vi "Access File Compress Database.vi"(8 "error in":errorcluster caption="error in (no error)", 11 "Access File Path":path caption="Access File Path (*.mdb)") -> (0 "error out":errorcluster)   [LabVIEW 2014]
panel:
  # "Input"
  # "Local"
  # "Output"
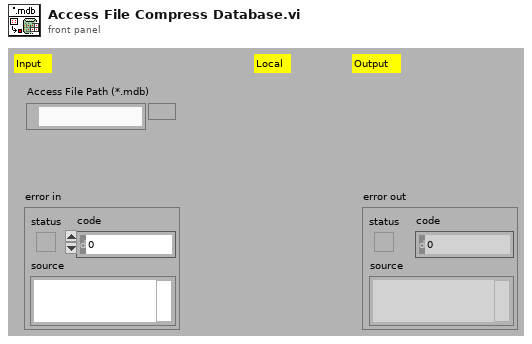
[diagram p1: front panel]
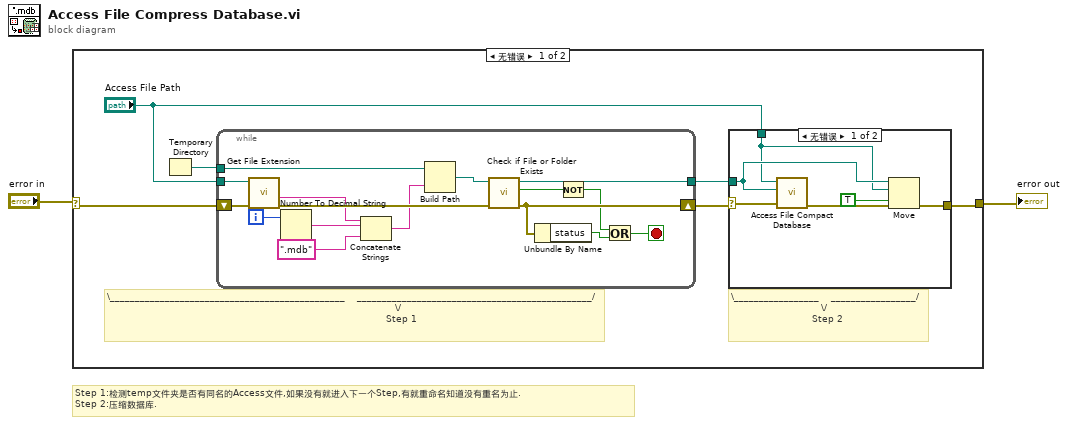
[diagram p0: block diagram]
diagram:
  # "Step 1:检测temp文件夹是否有同名的Access文件,如果没有就进入下一个Step,有就重命名知道没有重名为止.\nStep 2:压缩数据库."
  n1 = case shown="无错误" "error in" {
    selector: "error in" -> [w7 w32]
    tunnel: [w4 w32] -> w1
    frame No Error {
      # "\\_________________    _________________/\n                              \\/\n                           Step 2"
      # "\\_______________________________________________    _______________________________________________/\n                                                                                                \\/\n                                                                                             Step 1"
      n2 = Temporary Directory() -> (w8:path)
      n3 = while {
        tunnel: w8 -> [w21]
        shift-right: [w27] -> w6
        shift-left: w7 -> [w23]
        tunnel: [w28] -> w5
        tunnel: "Access File Path" -> [w24]
        i -> [w25]
        stop <- w31 stop-if-true
        n4 = call <vilib>:"Get File Extension.vi"("error in (no error)"=w23, "file"=w24) -> ("error out"=w20:errorcluster, "filename without extension"=w16:string)  [unwired: 6 in, 2 out]
        n5 = Number To Decimal String(number=w25) -> (decimal integer string=w22:string)  [unwired: 1 in]
        n6 = Concatenate Strings(w16, w22, ".mdb") -> (w19:string)
        n7 = Build Path(base path=w21, name or relative path=w19) -> (appended path=w18:path)
        n8 = call <vilib>:"Check if File or Folder Exists.vi"("error in (no error)"=w20, "path"=w18) -> ("error out"=w27:errorcluster, "file or folder exists?"=w29:bool, "dup path"=w28:path)  [unwired: 7 in]
        n9 = Unbundle By Name(w27) -> ("status"=w30:bool)
        n10 = Not(x=w29) -> (.not. x?=w26:bool)
        n11 = Or(x=w26, y=w30) -> (x .or. y?=w31:bool)
      }
      n12 = case shown="无错误" w6 {
        selector: w6 -> [w14 w15]
        tunnel: w5 -> [w12 _]
        tunnel: "Access File Path" -> [w11 _]
        tunnel: [w10 w15] -> w4
        frame No Error {
          n13 = call "Access File Compact Database.vi"("error in"=w14, "Destination Access File Path"=w12, "Source Access File Path"=w11) -> ("error out"=w13:errorcluster)  [unwired: 7 in, 1 out]
          n14 = Move(source path=w12, error in=w13, 9:TRUE ("overwrite (F)"), 10:w11) -> (error out=w10:errorcluster)  [unwired: 1 in, 2 out]
        }
        frame Error {
        }
      }
    }
    frame Error {
    }
  }
  "error out" <- w1
